vi "Send Control Mouse Up.vi"(0 "Message Enqueuer in":refnum<class "Message Enqueuer.lvclass">, 1 "Ctl Refnum":refnum<vi>, 2 "Use Label Text (F=Use Caption)":bool, 5 "Time":u32, 7 "Coords":T2, 9 "Button":u16, 11 "Mods":cluster{"Double Click":bool, "Menu Key":bool}, 12 "PlatMods":T1, 13 "Name (Get Text From Control)":string) -> (15 "error out":errorcluster)   [LabVIEW 2015, in "ActorAutoRegistration.lvlib" / "ControlMouseUpMsg.lvclass"]
doc: "<License>\nCopyright © 2017 Composed Systems, LLC | All rights reserved\nwww.composed.io\n\nAuthor: Ethan Stern <ethan.stern@composed.io>\n\nThis software is provided \"AS IS\" WITHOUT WARRANTIES, either express or implied, AND IS FOR EDUCATIONAL PURPOSES ONLY.\n</License>"
uses:
  ControlMouseUpMsg.lvclass
  <vilib>/ActorFramework/Message Enqueuer/Message Enqueuer.lvclass
  <vilib>/Utility/miscctls.llb/LVPoint32TypeDef.ctl
  ControlMouseUpMsg.lvclass/ControlMouseUpMsg.ctl
  EventDataMessage/EventDataMessage.lvclass
panel:
  in  "error in (no error)":errorcluster
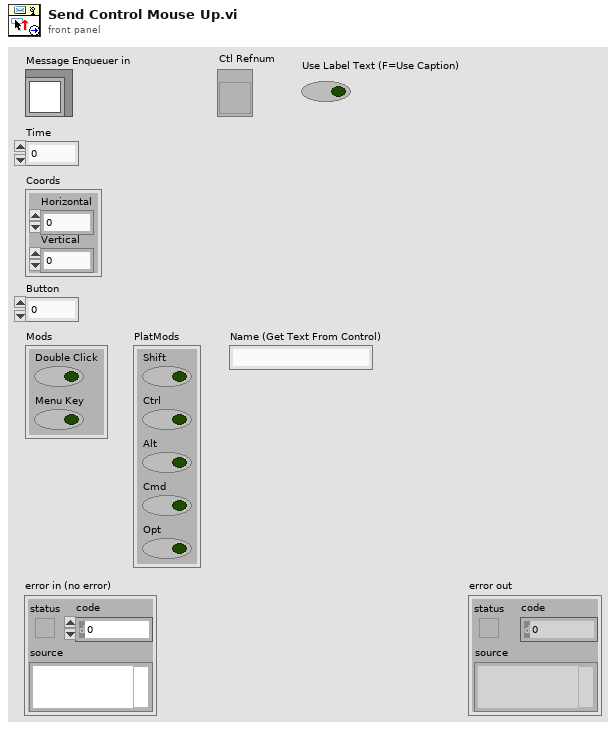
[diagram p1: front panel]
types:
  T1 = cluster{"Shift":bool, "Ctrl":bool, "Alt":bool, "Cmd":bool, "Opt":bool}
  T2 = typedef "LVPoint32TypeDef.ctl" = cluster{"Horizontal":i32, "Vertical":i32}
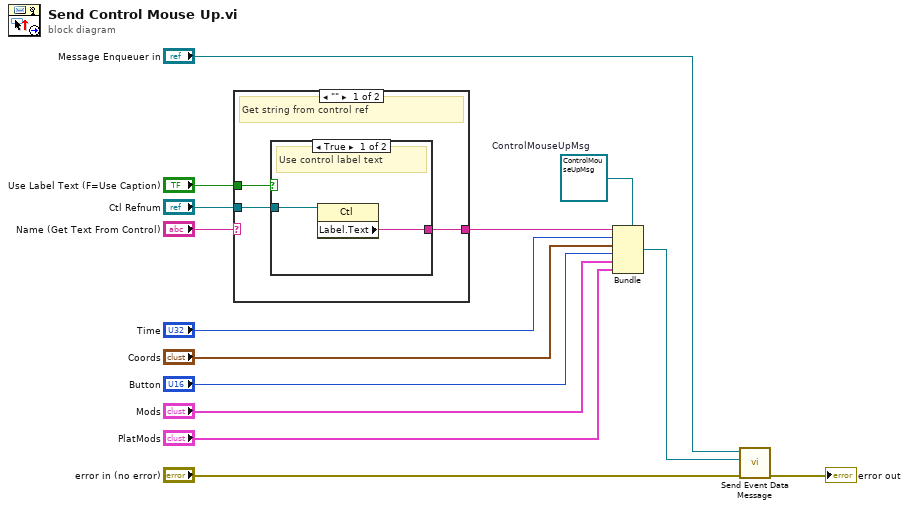
[diagram p0: block diagram]
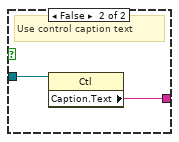
[diagram p2: hidden frame]
diagram:
  w14 = refnum<class "ControlMouseUpMsg.lvclass"> refnum  # ControlMouseUpMsg
  n1 = case shown="\"\"" "Name (Get Text From Control)" {
    selector: "Name (Get Text From Control)" -> [_ w22]
    tunnel: [w15 w22] -> w8
    tunnel: "Use Label Text (F=Use Caption)" -> [w17 _]
    tunnel: "Ctl Refnum" -> [w16 _]
    frame "" {
      # "Get string from control ref"
      n2 = case shown="True" w17 {
        tunnel: w16 -> [w19 w21]
        tunnel: [w18 w20] -> w15
        frame True {
          # "Use control label text"
          n3 = property class="Ctl"(reference=w19) -> ("Label.Text"=w18:string)  [unwired: 1 in, 2 out]
        }
        frame False {
          # "Use control caption text"
          n4 = property class="Ctl"(reference=w21) -> ("Caption.Text"=w20:string)  [unwired: 1 in, 2 out]
        }
      }
    }
    frame Default {
      # "Use string wired to input terminal"
    }
  }
  n5 = Bundle(cluster=w14, w8, "Time", "Coords", "Button", "Mods", "PlatMods") -> (w11:refnum<class "ControlMouseUpMsg.lvclass">)
  n6 = call "Send Event Data Message.vi"("error in (no error)"="error in (no error)", "EventDataMessage in"=w11, "Message Enqueuer in"="Message Enqueuer in") -> ("error out"=→"error out":errorcluster)  [unwired: 8 in]
